vi "LIA7230_read.vi"(4 "Range dual mode":u8(ring)=26 items=["N/A", "2nV", "5nV", "10nV", "20nV", "50nV", "100nV", "200nV", "500nV", "1µV", "2µV", "5µV", "10µV", "20µV", "50µV", "100µV", "200µV", "500µV", "1mV", "2mV", "5mV", "10mV", "20mV", "50mV", "100mV", "200mV", "500mV", "1V"], 6 "Reference Mode":bool, 7 "Range single mode":u8(ring)=26 items=["N/A", "2nV", "5nV", "10nV", "20nV", "50nV", "100nV", "200nV", "500nV", "1µV", "2µV", "5µV", "10µV", "20µV", "50µV", "100µV", "200µV", "500µV", "1mV", "2mV", "5mV", "10mV", "20mV", "50mV", "100mV", "200mV", "500mV", "1V"], 8 "error in (no error)":errorcluster, 9 "Input Mode":u16(ring)=1 items=["Inputs Grounded (test)", "A (Single-Ended Voltage)", "-B (Inverting Single Ended Voltage)", "A-B (Differential Voltage)", "AUX Input - Main Console", "B Current input - Wide Bandwidth", "B Current input - Low Noise"], 10 "Display Type":u16(ring)=5 items=["X %", "Y %", "X Calibrated", "Y Calibrated", "Mag %", "Mag Calibrated", "Phase Degrees", "Ratio", "Log Ratio", "ADC 1", "ADC 2", "ADC 3", "ADC 4", "Noise %", "Noise Calibrated", "Ref Frequency", "Equation 1", "Equation 2"], 11 "VISA session (for class)":refnum<visa-resource-name>) -> (0 "error out":errorcluster, 1 "Units":string="mV", 2 "Display":dbl=501.35 format="%.6f", 3 "VISA session (out)":refnum<visa-resource-name>, 5 "Overload":bool)   [LabVIEW 2019]
panel:
  # "Output"
  # "Dual"
  # "Single"
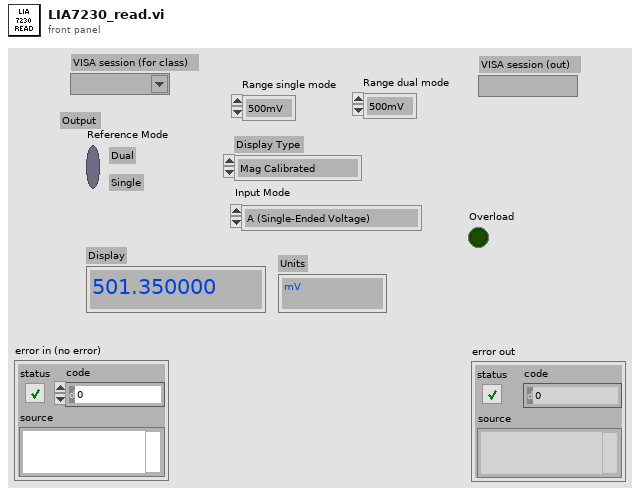
[diagram p1: front panel]
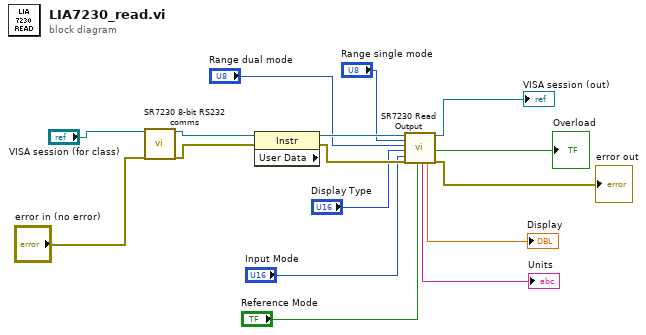
[diagram p0: block diagram]
diagram:
  n1 = call "SR7230 8-bit RS232 comms.vi"("VISA session (for class)"="VISA session (for class)", "error in (no error)"="error in (no error)") -> ("VISA session"=w16:refnum<visa-resource-name>, "error out"=w15:errorcluster)  [unwired: 16 in]
  n2 = property class="Instr" props=["User Data"](reference=w16, error in=w15) -> (reference out=w14:refnum<visa-resource-name>, error out=w13:errorcluster)  [unwired: 1 out]
  n3 = call "SR7230 Read Output.vi"("VISA session (for class)"=w14, "Range"="Range single mode", "Range 2"="Range dual mode", "Display Type"="Display Type", "error in (no error)"=w13, "Input Mode"="Input Mode", "Reference Mode"="Reference Mode") -> ("Units"=→"Units":string, "Display"=→"Display":dbl, "VISA session"=→"VISA session (out)":refnum<visa-resource-name>, "Overload"=→"Overload":bool, "error out"=→"error out":errorcluster)  [unwired: 4 in, 4 out]
